vi "Shooter_Begin.vi"() -> ()   [LabVIEW 2020]
uses:
  Shooter_Cluster.ctl
  Shooter_Control_States.ctl
  Subsystems/Turret/Turret_Cluster.ctl
  Subsystems/Turret/Turret_States.ctl
  Subsystems/Cowl/Cowl_Cluster.ctl
  Subsystems/Cowl/Cowl_States.ctl
  Subsystems/Flywheel/Flywheel_Cluster.ctl
  Subsystems/Flywheel/Flywheel_States.ctl
  Shooter_Globals.vi
  Globals/Turret_Globals.vi
  Globals/Cowl_Globals.vi
  Globals/Flywheel_Globals.vi
  Globals/FilePath_Globals.vi
  <vilib>/Utility/file.llb/Read Delimited Spreadsheet (DBL).vi
panel:
  out "all rows":dbl[][](array[numeric])
  out "appended path":path
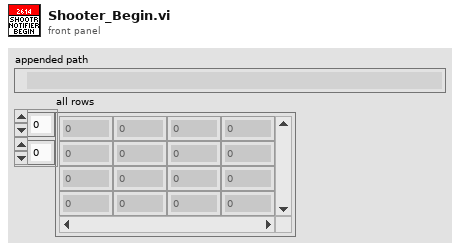
[diagram p1: front panel]
types:
  T1 = typedef "Flywheel_Cluster.ctl" = cluster{"Flywheel_Throttle":dbl, "Flywheel_Control_State":T2, "Parameter_1":dbl, "Parameter_2":dbl, "Auto_Notifier":refnum<notifier>, "Step":dbl, "Flywheel_Velocity_Goal":dbl, "Flywheel_On ":bool}
  T2 = typedef "Flywheel_States.ctl" = enum16{"No-Op", "Percent_Voltage", "Speed_Control", "Speed_Control_Manual", "Command_SpinUp", "Command_SpinUpAuto"}
  T3 = typedef "Cowl_Cluster.ctl" = cluster{"Cowl_Control_State":T4, "Manual_Cowl_Throttle":dbl, "Cowl_Goal_Angle":dbl}
  T4 = typedef "Cowl_States.ctl" = enum16{"Manual_%VBus", "GoToAngle", "No-Op", "GoToZero"}
  T5 = typedef "Turret_Cluster.ctl" = cluster{"Turret_Control_State":T6, "Manual_Speed":dbl, "Step":i32, "Parameter_1":dbl, "Parameter_2":dbl, "Parameter_3":dbl, "Auto_Notifier":refnum<notifier>, "Goal_Angle":dbl, "Camera_Goal_X":dbl}
  T6 = typedef "Turret_States.ctl" = enum16{"Manual_Percent_Voltage", "Auto-Target", "Command_TurnToPosition", "Command_Auto_Target", "GoToZero", "No-Op", "Test_Position_Control"}
  T7 = typedef "Shooter_Cluster.ctl" = cluster{"Control_State":T8, "Shooting?":bool, "UpperGoal?":bool, "Limelight?":bool, "Flywheel_%Vbus":dbl, "Cowl_%Vbus":dbl, "Turret_%Vbus":dbl, "Parameters":dbl[], "Auto_Notifier":refnum<notifier>, "Step":i32, "Zero_Turret":bool, "Puke?":bool}
  T8 = typedef "Shooter_Control_States.ctl" = enum16{"No-Op", "Limelight_Shooting", "Shoot_From_Pose", "Test", "Command_Shoot", "Turret_Cowl_Zero", "Manual", "Puke-Op"}
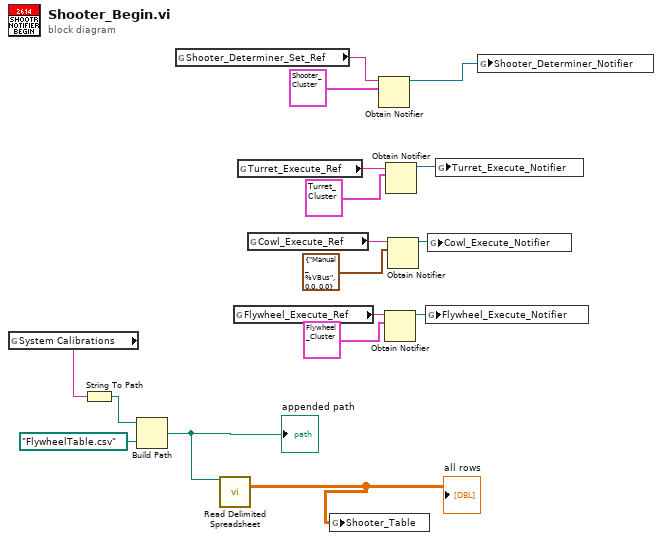
[diagram p0: block diagram]
diagram:
  n1 = global read "FilePath_Globals.vi" "System Calibrations"() -> (w2:string)
  n2 = String To Path(string=w2) -> (path=w1:path)
  n3 = Build Path(base path=w1, name or relative path=path "FlywheelTable.csv") -> (appended path=w4:path)
  "appended path" <- w4
  n4 = global read "Shooter_Globals.vi" "Shooter_Determiner_Set_Ref"() -> (w16:string)
  n5 = call-poly <vilib>:"Read Delimited Spreadsheet.vi"("file path (dialog if empty)"=w4) -> ("all rows"=w3:dbl[][])  [unwired: 9 in, 5 out]
  "all rows" <- w3
  n6 = global read "Flywheel_Globals.vi" "Flywheel_Execute_Ref"() -> (w7:string)
  n7 = global read "Turret_Globals.vi" "Turret_Execute_Ref"() -> (w14:string)
  n8 = global read "Cowl_Globals.vi" "Cowl_Execute_Ref"() -> (w10:string)
  n9 = global write "Shooter_Globals.vi" "Shooter_Table"(w3) -> ()
  n10 = Obtain Notifier(name (unnamed)=w16, notification data type=T7 {"Control_State"=enum."No-Op", "Shooting?"=FALSE, "UpperGoal?"=FALSE, "Limelight?"=FALSE, "Flywheel_%Vbus"=0.0, "Cowl_%Vbus"=0.0, "Turret_%Vbus"=0.0, "Parameters"=[], "Auto_Notifier"=refnum, "Step"=0, "Zero_Turret"=FALSE, "Puke?"=FALSE}) -> (notifier out=w17:refnum<notifier>)  [unwired: 2 in, 2 out]
  n11 = Obtain Notifier(name (unnamed)=w7, notification data type=T1 {"Flywheel_Throttle"=0.0, "Flywheel_Control_State"=enum."No-Op", "Parameter_1"=0.0, "Parameter_2"=0.0, "Auto_Notifier"=refnum, "Step"=0.0, "Flywheel_Velocity_Goal"=0.0, "Flywheel_On "=FALSE} ("Flywheel_Cluster")) -> (notifier out=w8:refnum<notifier>)  [unwired: 2 in, 2 out]
  n12 = Obtain Notifier(name (unnamed)=w14, notification data type=T5 {"Turret_Control_State"=enum."Manual_Percent_Voltage", "Manual_Speed"=0.0, "Step"=0, "Parameter_1"=0.0, "Parameter_2"=0.0, "Parameter_3"=0.0, "Auto_Notifier"=refnum, "Goal_Angle"=0.0, "Camera_Goal_X"=0.0} ("Turret_Cluster")) -> (notifier out=w12:refnum<notifier>)  [unwired: 2 in, 2 out]
  n13 = Obtain Notifier(name (unnamed)=w10, notification data type=T3 {"Cowl_Control_State"=enum."Manual_%VBus", "Manual_Cowl_Throttle"=0.0, "Cowl_Goal_Angle"=0.0} ("Cowl_Cluster")) -> (notifier out=w11:refnum<notifier>)  [unwired: 2 in, 2 out]
  n14 = global write "Flywheel_Globals.vi" "Flywheel_Execute_Notifier"(w8) -> ()
  n15 = global write "Cowl_Globals.vi" "Cowl_Execute_Notifier"(w11) -> ()
  n16 = global write "Turret_Globals.vi" "Turret_Execute_Notifier"(w12) -> ()
  n17 = global write "Shooter_Globals.vi" "Shooter_Determiner_Notifier"(w17) -> ()
